vi "dfd_Build String Line.vi"(7 "indent order":i32, 11 "string":string) -> (3 "string line":string)   [LabVIEW 2017, in "NI_DigFilter_Process.lvlib"]
uses:
  <vilib>/addons/Digital Filter Design/NI_DigFilter_Process.lvlib
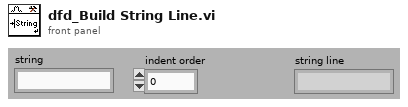
[diagram p1: front panel]
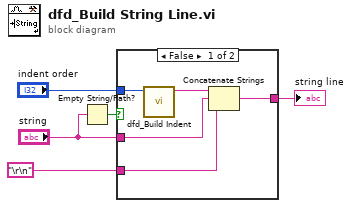
[diagram p0: block diagram]
diagram:
  n1 = Empty String/Path?(string/path="string") -> (empty?=w1:bool)
  n2 = case shown="False" w1 {
    tunnel: "indent order" -> [w10 _]
    tunnel: "string" -> [w8 _]
    tunnel: "\r\n" -> [w7 _]
    tunnel: [w6 _] -> w3
    frame False {
      n3 = call <vilib>:"dfd_Build Indent.vi"("indent order"=w10) -> ("tag indent"=w9:string)  [unwired: 10 out]
      n4 = Concatenate Strings(w9, w8, w7) -> (w6:string)
    }
    frame True {
    }
  }
  "string line" <- w3
